vi "ZLIB Open Zip__ogtk.vi"   [LabVIEW 2020]
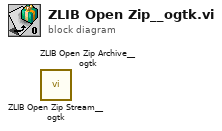
[diagram p0: block diagram]
diagram:
  n1 = call <userlib>:"ZLIB Open Zip Stream__ogtk.vi"() -> ()  [unwired: 5 in, 3 out]
  n2 = call <userlib>:"ZLIB Open Zip Archive__ogtk.vi"() -> ()  [unwired: 5 in, 3 out]
